vi "Thread Page GUID.vi"() -> (3 "Thread GUID":string="41c5f14b-093c-4be0-bff4-80a9437906d9")   [LabVIEW 2017, in "DSF Shared.lvlib"]
uses:
  DSF Shared.lvlib
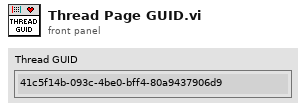
[diagram p1: front panel]
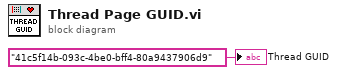
[diagram p0: block diagram]
diagram:
  "Thread GUID" <- "41c5f14b-093c-4be0-bff4-80a9437906d9" ("Data Sharing Framework")
